vi "Sample_02.vi"() -> ()   [LabVIEW 2018]
uses:
  <vilib>/Instr/_visa.llb/VISA Configure Serial Port (Instr).vi
panel:
  in  "(ml) 2":dbl=1.0
  in  "(ml)":dbl=1.0
  in  "Pump working wait time (Sec)":u32=5
  in  "Command wait time (Sec)":u32=2
  in  "VISA resource name 2":refnum<visa-resource-name>="COM5"
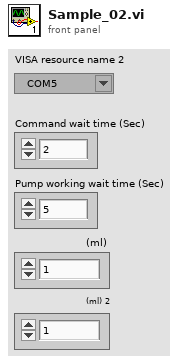
[diagram p1: front panel]
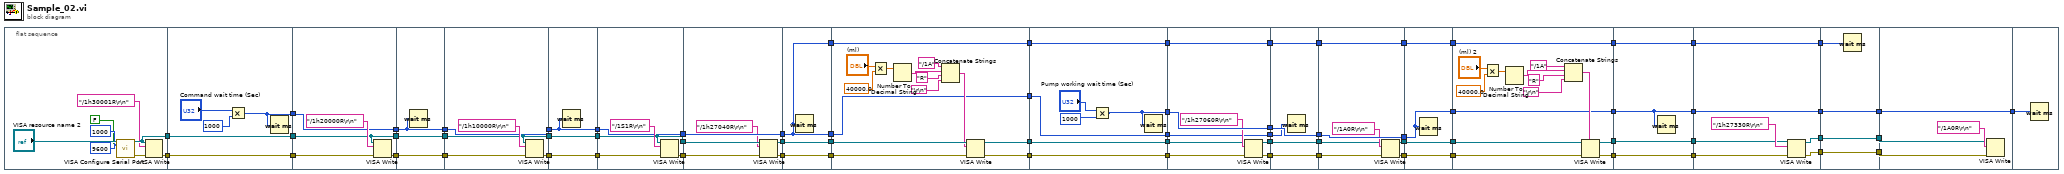
[diagram p0: block diagram]
diagram:
  n1 = flat-sequence {
    tunnel: [w72] -> w69
    tunnel: [w71] -> w68
    tunnel: w69 -> [w82]
    tunnel: w68 -> [w81]
    tunnel: [w82] -> w67
    tunnel: [w81] -> w66
    tunnel: [w78] -> w46
    tunnel: w67 -> [w85]
    tunnel: w66 -> [w86]
    tunnel: [w85] -> w64
    tunnel: [w84] -> w62
    tunnel: [w83] -> w47
    tunnel: w46 -> [w83]
    tunnel: [w90] -> w65
    tunnel: w64 -> [w90]
    tunnel: [w89] -> w63
    tunnel: w62 -> [w89]
    tunnel: w47 -> [w88]
    tunnel: [w88] -> w44
    tunnel: w65 -> [w92]
    tunnel: w63 -> [w94]
    tunnel: [w93] -> w60
    tunnel: [w92] -> w58
    tunnel: [w91] -> w45
    tunnel: w44 -> [w91]
    tunnel: [w98] -> w61
    tunnel: w60 -> [w98]
    tunnel: w58 -> [w97]
    tunnel: [w97] -> w57
    tunnel: w45 -> [w96]
    tunnel: [w96] -> w41
    tunnel: w61 -> [w102]
    tunnel: [w101] -> w59
    tunnel: w57 -> [w100]
    tunnel: [w100] -> w56
    tunnel: [w99] -> w42
    tunnel: w41 -> [w99]
    tunnel: w59 -> [w109]
    tunnel: w56 -> [w108]
    tunnel: [w107] -> w54
    tunnel: [w106] -> w52
    tunnel: [w105] -> w43
    tunnel: w42 -> [w105]
    tunnel: [w112] -> w55
    tunnel: w54 -> [w112]
    tunnel: [w111] -> w53
    tunnel: w52 -> [w111]
    tunnel: w43 -> [w110]
    tunnel: [w110] -> w33
    tunnel: [w110] -> w18
    tunnel: w55 -> [w126]
    tunnel: w53 -> [w125]
    tunnel: [w124] -> w50
    tunnel: [w123] -> w48
    tunnel: [w114] -> w34
    tunnel: w33 -> [w114]
    tunnel: [w113] -> w19
    tunnel: w18 -> [w113]
    tunnel: [w133] -> w51
    tunnel: w50 -> [w133]
    tunnel: [w132] -> w49
    tunnel: w48 -> [w132]
    tunnel: [w127] -> w40
    tunnel: [w131] -> w35
    tunnel: w34 -> [w131]
    tunnel: [w130] -> w20
    tunnel: w19 -> [w130]
    tunnel: w51 -> [w138]
    tunnel: w49 -> [w139]
    tunnel: [w141] -> w32
    tunnel: w40 -> [w141]
    tunnel: [w137] -> w31
    tunnel: [w136] -> w30
    tunnel: [w135] -> w29
    tunnel: w35 -> [w135]
    tunnel: [w134] -> w21
    tunnel: w20 -> [w134]
    tunnel: w32 -> [w146]
    tunnel: [w146] -> w38
    tunnel: w31 -> [w145]
    tunnel: [w145] -> w37
    tunnel: w30 -> [w144]
    tunnel: [w144] -> w36
    tunnel: w29 -> [w143]
    tunnel: [w142] -> w22
    tunnel: w21 -> [w142]
    tunnel: w38 -> [w153]
    tunnel: [w153] -> w39
    tunnel: w37 -> [w151]
    tunnel: w36 -> [w150]
    tunnel: [w149] -> w27
    tunnel: [w148] -> w25
    tunnel: [w147] -> w23
    tunnel: w22 -> [w147]
    tunnel: w39 -> [w154]
    tunnel: [w157] -> w28
    tunnel: w27 -> [w157]
    tunnel: [w156] -> w26
    tunnel: w25 -> [w156]
    tunnel: [w155] -> w24
    tunnel: w23 -> [w155]
    tunnel: [w154] -> w15
    tunnel: w28 -> [w163]
    tunnel: w26 -> [w162]
    tunnel: w24 -> [w158]
    tunnel: [w161] -> w17
    tunnel: [w160] -> w16
    tunnel: w15 -> [w160]
    tunnel: [w159] -> w13
    tunnel: [w158] -> w9
    tunnel: w17 -> [w174]
    tunnel: w16 -> [w172]
    tunnel: [w175] -> w14
    tunnel: w13 -> [w175]
    tunnel: [w174] -> w12
    tunnel: [w173] -> w10
    tunnel: w9 -> [w173]
    tunnel: [w172] -> w1
    tunnel: w14 -> [w181]
    tunnel: w12 -> [w180]
    tunnel: [w179] -> w11
    tunnel: w10 -> [w179]
    tunnel: [w178] -> w7
    tunnel: [w177] -> w5
    tunnel: [w176] -> w2
    tunnel: w1 -> [w176]
    tunnel: w11 -> [w186]
    tunnel: [w185] -> w8
    tunnel: w7 -> [w185]
    tunnel: [w184] -> w6
    tunnel: w5 -> [w184]
    tunnel: [w183] -> w3
    tunnel: w2 -> [w183]
    tunnel: w8 -> [w189]
    tunnel: w6 -> [w188]
    tunnel: [w187] -> w4
    tunnel: w3 -> [w187]
    tunnel: w4 -> [w191]
    frame #0 {
      n2 = call-poly "VISA Configure Serial Port"("VISA resource name"="VISA resource name 2", "timeout (10sec)"=u32 1000, "Enable Termination\nChar (T)"=FALSE ("Enable Termination\nChar (T)"), "baud rate (9600)"=u32 9600) -> ("VISA resource name out"=w72:refnum<visa-resource-name>, "error out"=w73:errorcluster)  [unwired: 10 in]
      n3 = VISA Write(VISA resource name=w72, write buffer="/1h30001R\r\n" ("string"), error in (no error)=w73) -> (error out=w71:errorcluster)  [unwired: 2 out]
    }
    frame #1 {
      n4 = Multiply(x="Command wait time (Sec)", y=u32 1000) -> (x*y=w78:u32)
      n5 = Wait (ms)(milliseconds to wait=w78) -> ()  [unwired: 1 out]
    }
    frame #2 {
      n6 = VISA Write(VISA resource name=w85, write buffer="/1h20000R\r\n" ("string"), error in (no error)=w86) -> (error out=w84:errorcluster)  [unwired: 2 out]
    }
    frame #3 {
      n7 = Wait (ms)(milliseconds to wait=w88) -> ()  [unwired: 1 out]
    }
    frame #4 {
      n8 = VISA Write(VISA resource name=w92, write buffer="/1h10000R\r\n" ("string"), error in (no error)=w94) -> (error out=w93:errorcluster)  [unwired: 2 out]
    }
    frame #5 {
      n9 = Wait (ms)(milliseconds to wait=w96) -> ()  [unwired: 1 out]
    }
    frame #6 {
      n10 = VISA Write(VISA resource name=w100, write buffer="/1S1R\r\n" ("string"), error in (no error)=w102) -> (error out=w101:errorcluster)  [unwired: 2 out]
    }
    frame #7 {
      n11 = VISA Write(VISA resource name=w108, write buffer="/1h27040R\r\n" ("string"), error in (no error)=w109) -> (VISA resource name out=w106:refnum<visa-resource-name>, error out=w107:errorcluster)  [unwired: 1 out]
    }
    frame #8 {
      n12 = Wait (ms)(milliseconds to wait=w110) -> ()  [unwired: 1 out]
    }
    frame #9 {
      n13 = Multiply(x="(ml)", y=40000.0) -> (x*y=w116:dbl)
      n14 = Number To Decimal String(number=w116) -> (decimal integer string=w119:string)  [unwired: 1 in]
      n15 = Concatenate Strings("/1A" ("string"), w119, "R" ("string"), "\r\n") -> (w115:string)
      n16 = VISA Write(VISA resource name=w125, write buffer=w115, error in (no error)=w126) -> (VISA resource name out=w123:refnum<visa-resource-name>, error out=w124:errorcluster)  [unwired: 1 out]
    }
    frame #10 {
      n17 = Multiply(x="Pump working wait time (Sec)", y=u32 1000) -> (x*y=w127:u32)
      n18 = Wait (ms)(milliseconds to wait=w127) -> ()  [unwired: 1 out]
    }
    frame #11 {
      n19 = VISA Write(VISA resource name=w139, write buffer="/1h27060R\r\n" ("string"), error in (no error)=w138) -> (VISA resource name out=w137:refnum<visa-resource-name>, error out=w136:errorcluster)  [unwired: 1 out]
    }
    frame #12 {
      n20 = Wait (ms)(milliseconds to wait=w143) -> ()  [unwired: 1 out]
    }
    frame #13 {
      n21 = VISA Write(VISA resource name=w151, write buffer="/1A0R\r\n" ("string"), error in (no error)=w150) -> (VISA resource name out=w149:refnum<visa-resource-name>, error out=w148:errorcluster)  [unwired: 1 out]
    }
    frame #14 {
      n22 = Wait (ms)(milliseconds to wait=w154) -> ()  [unwired: 1 out]
    }
    frame #15 {
      n23 = Multiply(x="(ml) 2", y=40000.0) -> (x*y=w170:dbl)
      n24 = Number To Decimal String(number=w170) -> (decimal integer string=w168:string)  [unwired: 1 in]
      n25 = Concatenate Strings("/1A" ("string"), w168, "R" ("string"), "\r\n") -> (w171:string)
      n26 = VISA Write(VISA resource name=w163, write buffer=w171, error in (no error)=w162) -> (VISA resource name out=w159:refnum<visa-resource-name>, error out=w161:errorcluster)  [unwired: 1 out]
    }
    frame #16 {
      n27 = Wait (ms)(milliseconds to wait=w172) -> ()  [unwired: 1 out]
    }
    frame #17 {
      n28 = VISA Write(VISA resource name=w181, write buffer="/1h27330R\r\n" ("string"), error in (no error)=w180) -> (VISA resource name out=w178:refnum<visa-resource-name>, error out=w177:errorcluster)  [unwired: 1 out]
    }
    frame #18 {
      n29 = Wait (ms)(milliseconds to wait=w186) -> ()  [unwired: 1 out]
    }
    frame #19 {
      n30 = VISA Write(VISA resource name=w189, write buffer="/1A0R\r\n" ("string"), error in (no error)=w188) -> ()  [unwired: 3 out]
    }
    frame #20 {
      n31 = Wait (ms)(milliseconds to wait=w191) -> ()  [unwired: 1 out]
    }
  }
